vi "RPC Method ni_measurements_v1_MeasurementService_Measure Logic.vi"(8 "error in":errorcluster, 11 "gRPCid in":T1) -> (0 "error out":errorcluster)   [LabVIEW 2020, in "LoadRegulation.lvlib" / "MeasurementService.lvclass"]
uses:
  MeasurementService.lvclass/MeasurementService.ctl
  MeasurementService.lvclass
  b0ad159f-8a6c-4803-bb9d-e65e58ffa1c4.vi
  3d8d31dd-6022-44d1-aec6-106d91e19b82.vi
  LoadRegulation.lvlib
  Measurement Configuration.ctl
  <vilib>/gRPC/LabVIEW gRPC Library/Server API/typeDefs/gRPC Status Code.ctl
  <vilib>/gRPC/LabVIEW gRPC Library/gprc-lvsupport-release.lvlib
  <vilib>/gRPC/LabVIEW gRPC Library/Server API/typeDefs/grpcId.ctl
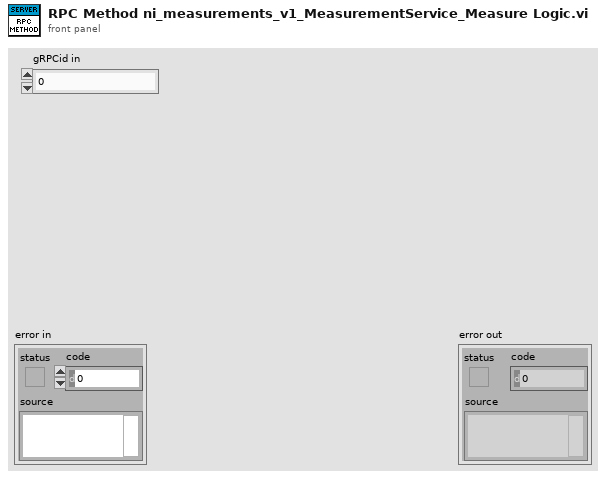
[diagram p1: front panel]
types:
  T1 = typedef "gprc-lvsupport-release.lvlib/grpcId.ctl" = u64
  T2 = typedef "LoadRegulation.lvlib/Measurement Configuration.ctl" = cluster{"Input Voltage in V":dbl, "Nominal Output Voltage in V":dbl, "Start":dbl, "Stop":dbl, "Step":dbl, "Input SMU":string, "Load SMU":string, "Input DMM":string, "Load DMM":string}
  T3 = typedef "LoadRegulation.lvlib/ni_measurements_v1_MeasureRequest.ctl" = cluster{"configuration_parameters":T4}
  T4 = typedef "LoadRegulation.lvlib/google_protobuf_Any.ctl" = cluster{"type_url":string, "value":u8[]}
  T5 = typedef "LoadRegulation.lvlib/Measurement Results.ctl" = cluster{"Load Regulation (%)":dbl, "Load Regulation (mV/mA)":dbl, "Test Results.Load Current in A":dbl[], "Output Voltage in V":dbl[]}
  T6 = typedef "gprc-lvsupport-release.lvlib/gRPC Status Code.ctl" = enum16{"OK", "CANCELLED", "UNKNOWN", "INVALID_ARGUMENT", "DEADLINE_EXCEEDED", "NOT_FOUND", "ALREADY_EXISTS", "PERMISSION_DENIED", "RESOURCE_EXHAUSTED", "FAILED_PRECONDITION", "ABORTED", "OUT_OF_RANGE", "UNIMPLEMENTED", "INTERNAL", "UNAVAILABLE", "DATA_LOSS", "UNAUTHENTICATED"}
  T7 = typedef "gprc-lvsupport-release.lvlib/Any.ctl" = cluster{"Type Url":string, "Bytes":u8[]}
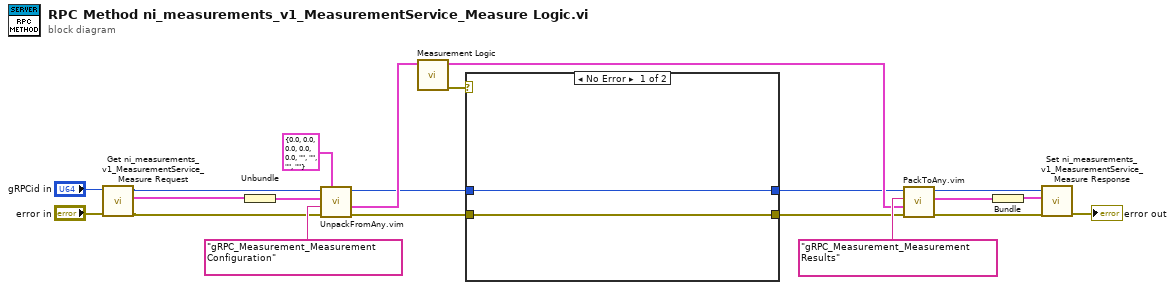
[diagram p0: block diagram]
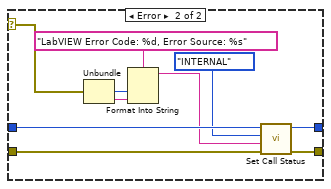
[diagram p2: hidden frame]
diagram:
  n1 = call "Get ni_measurements_v1_MeasurementService_Measure Request.vi"("error in (no error)"="error in", "gRPCid in"="gRPCid in") -> ("error out"=w14:errorcluster, "Message Data"=w15:T3, "gRPCid out"=w13:T1)  [unwired: 7 in]
  n2 = Unbundle(w15) -> ("configuration_parameters"=w21:T4)
  n3 = call "UnpackFromAny.vim"("Data Type"=T2 {"Input Voltage in V"=0.0, "Nominal Output Voltage in V"=0.0, "Start"=0.0, "Stop"=0.0, "Step"=0.0, "Input SMU"="", "Load SMU"="", "Input DMM"="", "Load DMM"=""} ("Measurement Configuration"), "error in (no error)"=w14, "Message Type"="gRPC_Measurement_Measurement Configuration", "Any"=w21, "gRPCid in"=w13) -> ("error out"=w5:errorcluster, "Unpacked Value"=w17:T2, "gRPCid"=w3:u64)  [unwired: 4 in]
  n4 = call "Measurement Logic.vi"("Measurement Configuration"=w17) -> ("error out"=w2:errorcluster, "Measurement Results"=w18:T5)  [unwired: 9 in]
  n5 = case shown="No Error" w2 {
    selector: w2 -> [_ w33]
    tunnel: w3 -> [w23 w32]
    tunnel: [w23 w31] -> w1
    tunnel: w5 -> [w22 w29]
    tunnel: [w22 w30] -> w4
    frame No Error {
    }
    frame Error {
      n6 = Unbundle(w33) -> ("code"=w27:i32, "source"=w26:string)  [unwired: 1 out]
      n7 = Format Into String(format string="LabVIEW Error Code: %d, Error Source: %s", w27, w26) -> (resulting string=w24:string)  [unwired: 2 in, 1 out]
      n8 = call <vilib>:"Set Call Status.vi"("error in (no error)"=w29, "Details"=w24, "Status Code"=gRPC_Status_Code."INTERNAL", "gRCP ID"=w32) -> ("error out"=w30:errorcluster, "gRCP ID Out"=w31:T1)  [unwired: 6 in]
    }
  }
  n9 = call "PackToAny.vim"("error in (no error)"=w4, "Data To Pack"=w18, "Message Type"="gRPC_Measurement_Measurement Results", "gRPCid in"=w1) -> ("error out"=w9:errorcluster, "Any"=w11:T7, "gRPCid"=w12:u64)  [unwired: 5 in]
  n10 = Bundle("Any"=w11) -> (w10:cluster{"Any":T7})  [unwired: 1 in]
  n11 = call "Set ni_measurements_v1_MeasurementService_Measure Response.vi"("error in (no error)"=w9, "Message Data"=w10, "gRPCid in"=w12) -> ("error out"=→"error out":errorcluster)  [unwired: 8 in]
